vi "Process Data.vi"(8 "error in (no error)":errorcluster, 10 "Upper Frequency Cutoff":dbl, 11 "Raw Data":dbl[][](array[numeric])) -> (0 "error out":errorcluster, 2 "Altitude":dbl[][](array[numeric]), 3 "Processed Data":dbl[][](array[numeric]))   [LabVIEW 2013]
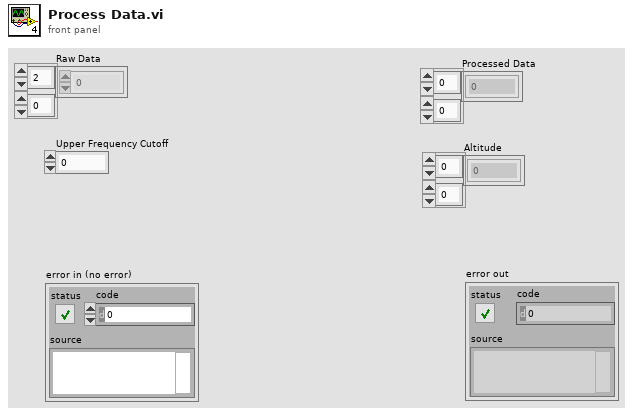
[diagram p1: front panel]
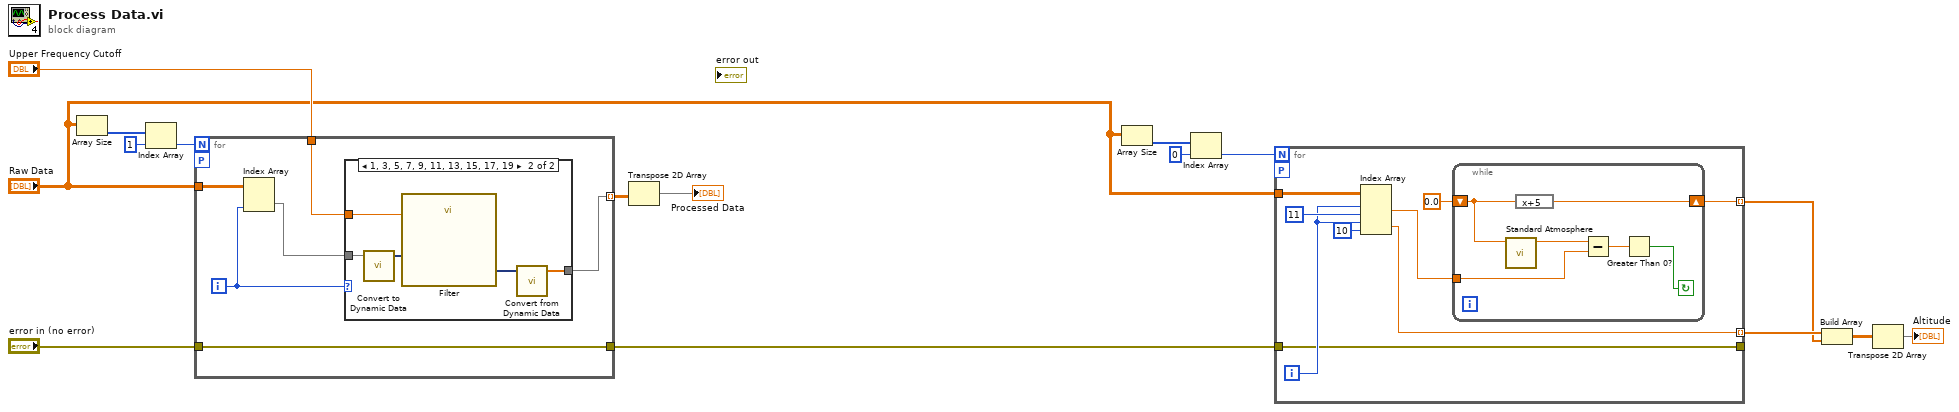
[diagram p0: block diagram]
diagram:
  n1 = Array Size(array="Raw Data") -> (size(s)=w16:i32[])
  n2 = Index Array(array=w16, index=1) -> (element=w14:i32)
  n3 = for {
    N: w14 -> [_]
    tunnel: [w22] -> w13 mode=indexing
    tunnel: "Raw Data" -> [w21]
    tunnel: "Upper Frequency Cutoff" -> [w18]
    tunnel: "error in (no error)" -> [w17]
    workers-P: _ -> [_]
    tunnel: [w17] -> w10
    i -> [w20]
    n4 = Index Array(array=w21, index (col)=w20) -> (element=w19:dbl[])  [unwired: 1 in]
    n5 = case shown="1, 3, 5, 7, 9, 11, 13, 15, 17, 19" w20 {
      tunnel: w19 -> [w23 w28]
      tunnel: [w23 w25] -> w22
      tunnel: w18 -> [_ w24]
      frame 0, Default {
      }
      frame 1, 3, 5, 7, 9, 11, 13, 15, 17, 19 {
        n6 = call "Convert to Dynamic Data"("Array"=w28) -> ("Dynamic Data Type"=w27:dynamicdata)  [unwired: 3 in]
        n7 = call "Filter"("Lower Cut-Off"=w24, "Signal"=w27) -> ("Filtered Signal"=w26:dynamicdata)  [unwired: 8 in, 1 out]
        n8 = call "Convert from Dynamic Data"("Dynamic Data Type"=w26) -> ("Array"=w25:dbl[])  [unwired: 3 in]
      }
    }
  }
  n9 = Transpose 2D Array(2D array=w13) -> (transposed array=→"Processed Data":dbl[][])
  n10 = Array Size(array="Raw Data") -> (size(s)=w9:i32[])
  n11 = Index Array(array=w9, index=0) -> (element=w7:i32)
  n12 = for {
    N: w7 -> [_]
    tunnel: "Raw Data" -> [w37]
    tunnel: w10 -> [w30]
    tunnel: [w34] -> w1 mode=indexing
    workers-P: _ -> [_]
    tunnel: [w29] -> w4 mode=indexing
    tunnel: [w30] -> _
    i -> [w33]
    n13 = Index Array(array=w37, index (row) #1=w33, index (col) #1=11 ("disabled index (col)"), index (row) #2=w33, index (col) #2=10 ("disabled index (col)")) -> (element #1=w31:dbl, element #2=w29:dbl)
    n14 = while {
      shift-right: [w39] -> w34
      shift-left: 0.0 -> [w38]
      tunnel: w31 -> [w41]
      stop <- w43 continue-if-true
      n15 = call "Standard Atmosphere.vi"("Altitude (m)"=w38) -> ("Pressure (Pa)"=w42:dbl)  [unwired: 7 in, 3 out]
      n16 = expression code="x+5"(w38) -> (w39:dbl)
      n17 = Subtract(x=w42, y=w41) -> (x-y=w40:dbl)
      n18 = Greater Than 0?(x=w40) -> (x > 0?=w43:bool)
    }
  }
  n19 = Build Array(w4, w1) -> (w3:dbl[][])
  n20 = Transpose 2D Array(2D array=w3) -> (transposed array=→"Altitude":dbl[][])
